vi "抽奖程序.vi"() -> ()   [LabVIEW 2017]
panel:
  in  "已经中奖的人":string[](array[string])
  in  "开始":bool
  out "中奖者":string
  in  "抽奖样本":string[](array[string])
  out "中奖者序号":dbl
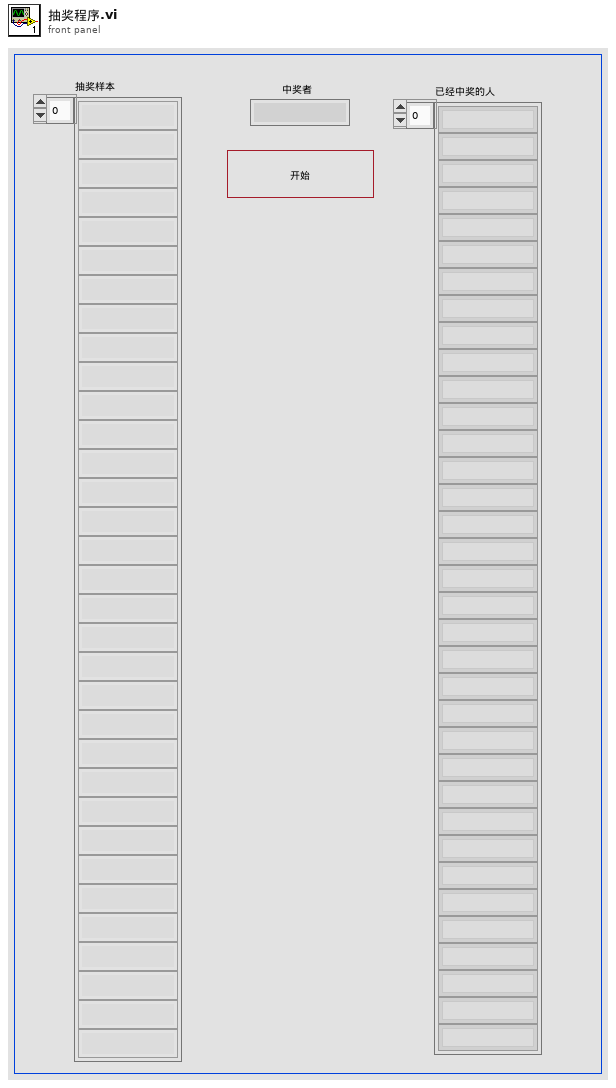
[diagram p1: front panel]
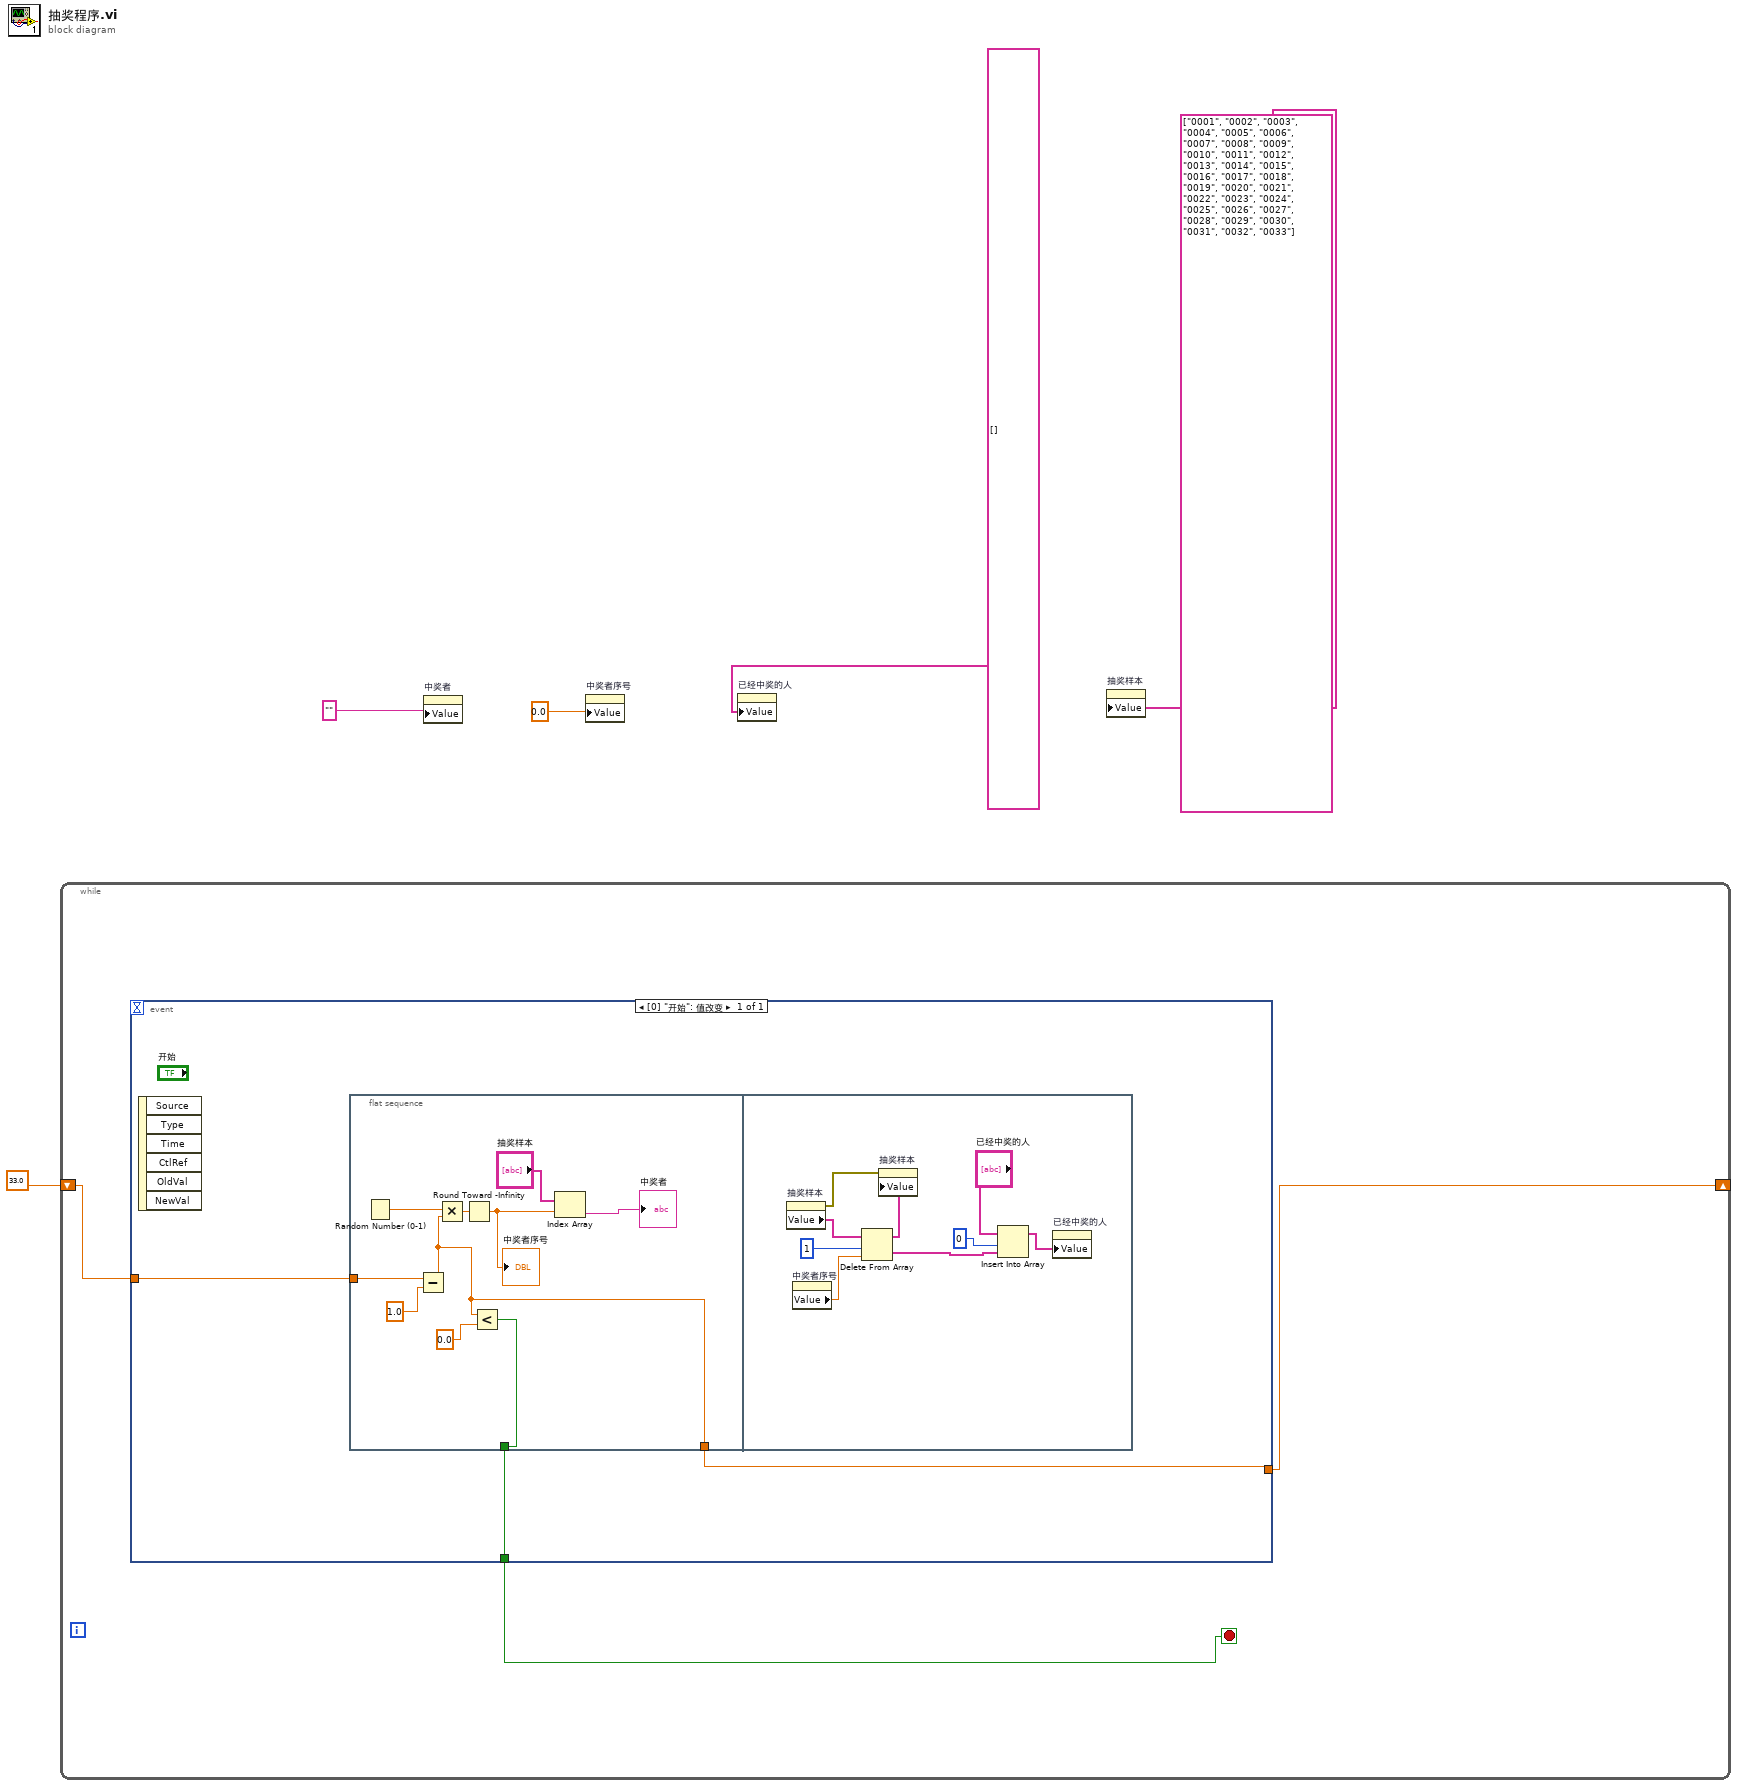
[diagram p0: block diagram]
diagram:
  n1 = while {
    shift-right: [w7] -> _
    shift-left: 33.0 -> [w8]
    stop <- w6 stop-if-true
    n2 = event shown="[0] \"开始\": 值改变" {
      selector: _ -> [_]
      dyn-events: _ -> [_]
      timeout: _ -> [_]
      tunnel: w8 -> [w11]
      tunnel: [w10] -> w7
      tunnel: [w9] -> w6
      event "开始": Value Change {
        n3 = event-data() -> ()  [unwired: 1 in, 6 out]
        n4 = flat-sequence {
          tunnel: [w12] -> _
          tunnel: w11 -> [w14]
          tunnel: [w13] -> w10
          tunnel: [w12] -> w9
          frame #0 {
            n5 = Random Number (0-1)() -> (number: 0 to 1=w17:dbl)
            n6 = Subtract(x=w14, y=1.0) -> (x-y=w13:dbl)
            n7 = Multiply(x=w17, y=w13) -> (x*y=w20:dbl)
            n8 = Round Toward -Infinity(1:w20) -> (0:w21:dbl)
            "中奖者序号" <- w21
            n9 = Less?(x=w13, y=0.0) -> (x < y?=w12:bool)
            n10 = Index Array(array="抽奖样本", index=w21) -> (element=→"中奖者":string)
          }
          frame #1 {
            n11 = property on="抽奖样本" class="Arr (严格)"() -> (error out=w22:errorcluster, "Value"=w29:string[])  [unwired: 2 in, 1 out]
            n12 = property on="中奖者序号" class="DigNum (严格)"() -> ("Value"=w30:dbl)  [unwired: 2 in, 2 out]
            n13 = Delete From Array(array=w29, length=1, index=w30) -> (deleted portion=w25:string[], array with subset deleted=w23:string[])
            n14 = property on="抽奖样本" class="Arr (严格)"(error in=w22, "Value"=w23) -> ()  [unwired: 1 in, 2 out]
            n15 = Insert Into Array(array="已经中奖的人", index=0, new element=w25) -> (w24:string[])
            n16 = property on="已经中奖的人" class="Arr (严格)"("Value"=w24) -> ()  [unwired: 2 in, 2 out]
          }
        }
      }
    }
  }
  n17 = property on="中奖者" class="Str"("Value"="") -> ()  [unwired: 2 in, 2 out]
  n18 = property on="中奖者序号" class="DigNum (严格)"("Value"=0.0) -> ()  [unwired: 2 in, 2 out]
  n19 = property on="已经中奖的人" class="Arr (严格)"("Value"=string[] [] ("数组")) -> ()  [unwired: 2 in, 2 out]
  n20 = property on="抽奖样本" class="Arr (严格)"("Value"=string[] ["0001", "0002", "0003", "0004", "0005", "0006", "0007", "0008", "0009", "0010", "0011", "0012", "0013", "0014", "0015", "0016", "0017", "0018", "0019", "0020", "0021", "0022", "0023", "0024", "0025", "0026", "0027", "0028", "0029", "0030", "0031", "0032", "0033"] ("所有人的学号")) -> ()  [unwired: 2 in, 2 out]
